vi "2.5.-Análisis Matricial de una Imagen.vi"() -> ()   [LabVIEW 2020]
panel:
  out "R después del filtro":u32
  in  "Boolean array":bool[](array[boolean])
  out "R":u8
  out "Color Box":u32(colorbox)
  out "2D Picture 2":picture
  out "2D Picture":picture
  in  "Path":path
  # "di_cer0 - Visión Artificial - LabVIEW"
  # "El VI lo que hace es determinar en cada pixel el nivel de gris e irlo mostrando en color de gris, valor numérico y array booleano, donde su bit más significativo es el de hasta abajo."
  # "Lo que pasa cuando desactivamos un bit del array es que se le resta una potencia de 2, yendo de 0 a 7  al valor de gris de salida, por eso es que con los primeros bits no es muy visible la diferencia, pero ya activando 5 bits del array, se empieza a ver capas de grises."
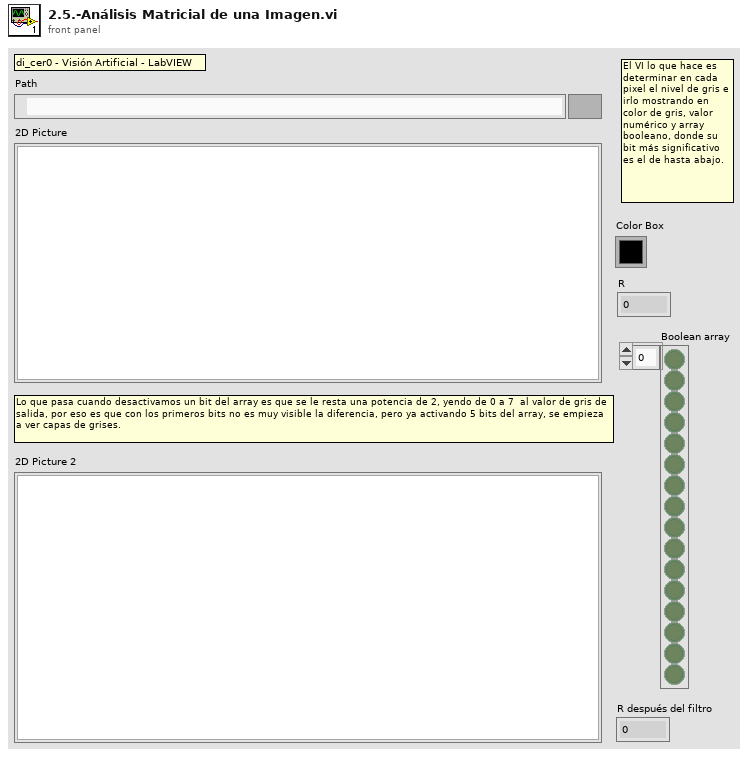
[diagram p1: front panel]
types:
  T1 = typedef "imagedata.ctl" = cluster{"image type":i32, "image depth":i32, "image":u8[], "mask":u8[], "colors":u32[], "Rectangle":cluster{"left":i16, "top":i16, "right":i16, "bottom":i16}}
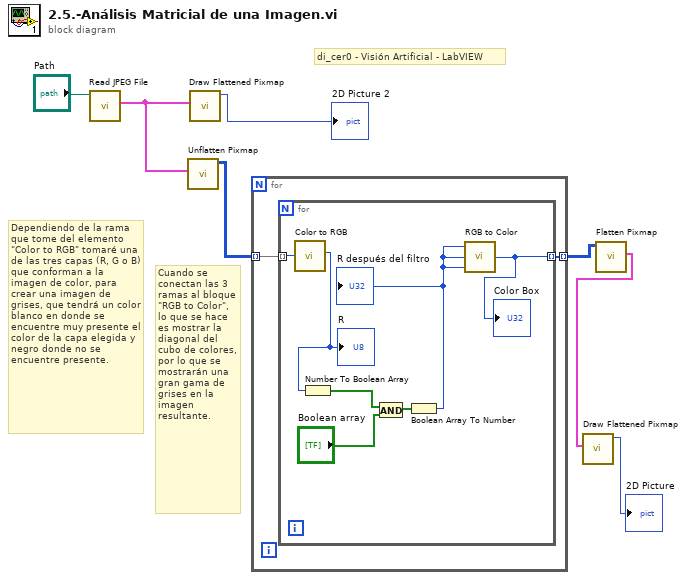
[diagram p0: block diagram]
diagram:
  # "di_cer0 - Visión Artificial - LabVIEW"
  # "Cuando se conectan las 3 ramas al bloque \"RGB to Color\", lo que se hace es mostrar la diagonal del cubo de colores, por lo que se mostrarán una gran gama de grises en la imagen resultante."
  # "Dependiendo de la rama que tome del elemento \"Color to RGB\" tomaré una de las tres capas (R, G o B) que conforman a la imagen de color, para crear una imagen de grises, que tendrá un color blanco en donde se encuentre muy presente el color de la capa elegida y negro donde no se encuentre presente."
  n1 = call <vilib>:"Read JPEG File.vi"("path to JPEG file"="Path") -> ("image data"=w6:T1)  [unwired: 8 in, 2 out]
  n2 = call <vilib>:"Unflatten Pixmap.vi"("image data"=w6) -> ("24-bit pixmap"=w5:u32[][])  [unwired: 4 in, 6 out]
  n3 = call <vilib>:"Draw Flattened Pixmap.vi"("image data"=w6) -> ("new picture"=→"2D Picture 2":picture)  [unwired: 8 in]
  n4 = for {
    tunnel: w5 -> [w9] mode=indexing
    tunnel: [w8] -> w4 mode=indexing
    n5 = for {
      tunnel: w9 -> [w16] mode=indexing
      tunnel: [w15] -> w8 mode=indexing
      n6 = call <vilib>:"Color to RGB.vi"("Color"=w16) -> ("R"=w14:u8)  [unwired: 3 out]
      "R" <- w14
      n7 = Number To Boolean Array(number=w14) -> (Boolean array=w13:bool[])
      n8 = And(x=w13, y="Boolean array") -> (x .and. y?=w11:bool[])
      n9 = Boolean Array To Number(Boolean array=w11) -> (number=w10:u32)
      "R después del filtro" <- w10
      n10 = call <vilib>:"RGB to Color.vi"("B"=w10, "G"=w10, "R"=w10) -> ("Color"=w15:u32)
      "Color Box" <- w15
    }
  }
  n11 = call <vilib>:"Flatten Pixmap.vi"("24-bit pixmap"=w4) -> ("image data"=w3:T1)  [unwired: 10 in]
  n12 = call <vilib>:"Draw Flattened Pixmap.vi"("image data"=w3) -> ("new picture"=→"2D Picture":picture)  [unwired: 8 in]
